vi "CheckIfCoordAreInElement.vi"(8 "error in (no error)":errorcluster, 10 "Coords":T1, 11 "Array in":refnum<vi>) -> (0 "error out":errorcluster, 3 "in element?":bool)   [LabVIEW 2023]
doc: "This VI checks if vertical coordinates fall within the image element of an image array."
uses:
  <vilib>/Utility/miscctls.llb/LVPoint32TypeDef.ctl
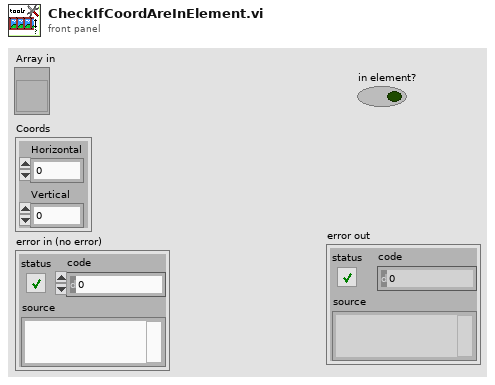
[diagram p1: front panel]
types:
  T1 = typedef "LVPoint32TypeDef.ctl" = cluster{"Horizontal":i32, "Vertical":i32}
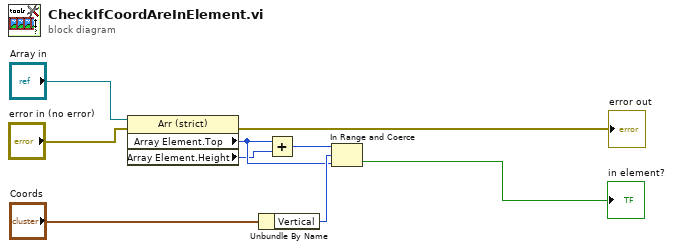
[diagram p0: block diagram]
diagram:
  n1 = property on="Property Node" class="Arr (strict)"(reference="Array in", error in="error in (no error)") -> (error out=→"error out":errorcluster, "Array Element.Top"=w6:i32, "Array Element.Height"=w5:u32)  [unwired: 1 out]
  n2 = Unbundle By Name("Coords") -> ("Vertical"=w8:i32)
  n3 = Add(x=w6, y=w5) -> (x+y=w7:u32)
  n4 = In Range and Coerce(upper limit=w7, x=w8, lower limit=w6) -> (In Range?=→"in element?":bool)  [unwired: 1 out]
